vi "Server_test_2.vi"() -> ()   [LabVIEW 2021]
panel:
  in  "Event":string
  out "Array":dbl[][](array[numeric])
  out "data string":string
  out "Array of element extracted\nfrom the array depending on \nthe coordinates given":dbl[](array[numeric])
  out "length":string
  out "Iteration":i32
  out "Command\nreceived":string
  out "error out":errorcluster
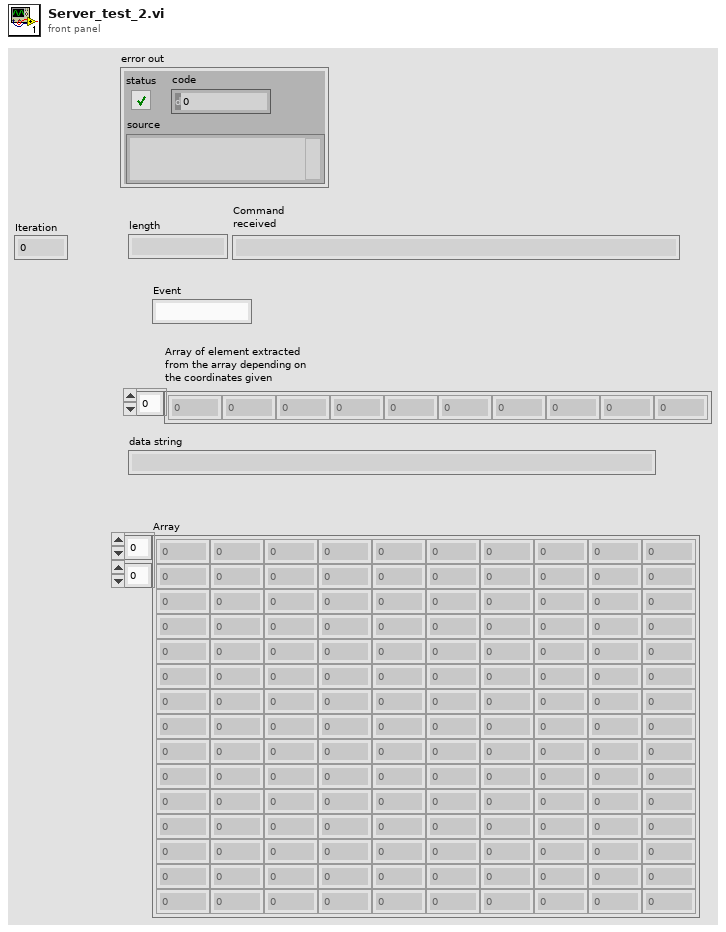
[diagram p1: front panel]
types:
  T1 = enum16{"big-endian, network order", "native, host order", "little-endian"}
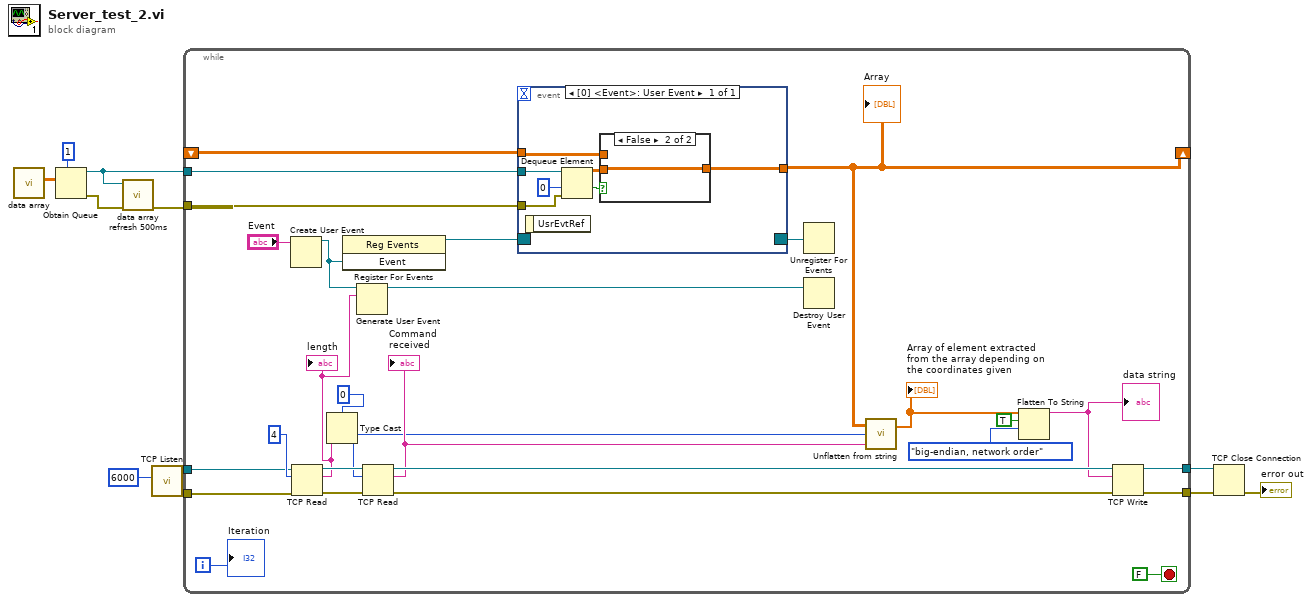
[diagram p0: block diagram]
diagram:
  n1 = call "data array.vi"() -> ("Array"=w10:dbl[][])  [unwired: 11 in]
  n2 = Obtain Queue(max queue size (-1, unlimited)=1, element data type=w10) -> (queue out=w9:refnum<queue>, error out=w8:errorcluster)  [unwired: 3 in, 1 out]
  n3 = call "data array refresh 500ms.vi"("error in (no error)"=w8, "queue out"=w9) -> ()  [unwired: 10 in]
  n4 = call <vilib>:"TCP Listen.vi"("port"=u16 6000) -> ("error out"=w2:errorcluster, "connection ID"=w1:refnum<k5>)  [unwired: 6 in, 3 out]
  n5 = while {
    tunnel: w9 -> [w14]
    tunnel: w8 -> [w13]
    tunnel: [w32] -> w5
    tunnel: [w31] -> w4
    tunnel: w2 -> [w30]
    tunnel: w1 -> [w29]
    shift-right: [w12] -> _
    shift-left: _ -> [w15]
    i -> [w34]
    stop <- FALSE stop-if-true
    n6 = Create User Event(user event datatype="Event") -> (user event=w18:refnum<user-event>)  [unwired: 1 in, 1 out]
    n7 = TCP Read(connection ID=w29, bytes to read=4, error in (no error)=w30) -> (connection ID out=w38:refnum<k5>, data out=w11:string, error out=w37:errorcluster)  [unwired: 2 in]
    "length" <- w11
    n8 = Type Cast(type=0, x=w11) -> (*(type *) &x=w22:i32)
    n9 = register-events(w18) -> (reference out=w19:refnum<event-registration>)  [unwired: 2 in, 1 out]
    n10 = Generate User Event(user event=w18, event data cluster=w11) -> (user event out=w16:refnum<user-event>)  [unwired: 2 in, 1 out]
    n11 = TCP Read(connection ID=w38, bytes to read=w22, error in (no error)=w37) -> (connection ID out=w28:refnum<k5>, data out=w23:string, error out=w27:errorcluster)  [unwired: 2 in]
    "Command\nreceived" <- w23
    n12 = event shown="[0] <Event>: User Event" {
      selector: w19 -> [_]
      dyn-events: [_] -> w17
      timeout: _ -> [_]
      tunnel: w15 -> [w43]
      tunnel: w14 -> [w42]
      tunnel: w13 -> [w40]
      tunnel: [w39] -> w12
      event User Event {
        n13 = event-data() -> ()  [unwired: 1 in, 1 out]
        n14 = Dequeue Element(queue=w42, timeout in ms (-1)=0, error in (no error)=w40) -> (element=w45:dbl[][], timed out?=w44:bool)  [unwired: 2 out]
        n15 = case shown="False" w44 {
          tunnel: w45 -> [_ w47]
          tunnel: w43 -> [w46 _]
          tunnel: [w46 w47] -> w39
          frame True {
          }
          frame False {
          }
        }
      }
    }
    "Array" <- w12
    n16 = Unregister For Events(event registration refnum=w17) -> ()  [unwired: 1 in, 1 out]
    n17 = Destroy User Event(user event=w16) -> ()  [unwired: 1 in, 1 out]
    n18 = call "Unflatten from string.vi"("Input string"=w23, "Number of coordinates to extract"=w22, "Array"=w12) -> ("Array of element extracted\nfrom the data array depending \non the coordinates given"=w21:dbl[])
    "Array of element extracted\nfrom the array depending on \nthe coordinates given" <- w21
    n19 = Flatten To String(anything=w21, prepend array or string size? (T)=TRUE, byte order (0:big-endian, network order)=T1."big-endian, network order") -> (data string=w24:string)  [unwired: 1 in, 2 out]
    "data string" <- w24
    n20 = TCP Write(connection ID=w28, data in=w24, error in (no error)=w27) -> (connection ID out=w31:refnum<k5>, error out=w32:errorcluster)  [unwired: 1 in, 1 out]
    "Iteration" <- w34
  }
  n21 = TCP Close Connection(connection ID=w4, error in (no error)=w5) -> (error out=→"error out":errorcluster)  [unwired: 1 in, 1 out]
